vi "Counter - Read Encoder (Continuous Clock).vi"() -> ()   [LabVIEW 2017]
doc: "This example demonstrates how to use a counter input along with an external clock to continually sample the angular position measured from an encoder.\n\nFor instructions on how to connect your signals to the DAQ device, refer to your device documentation."
uses:
  <vilib>/Utility/error.llb/DialogType.ctl
  <vilib>/DAQmx/read.llb/DAQmx Read (Counter 1D DBL 1Chan NSamp).vi
  <vilib>/DAQmx/read.llb/DAQmx Read (Analog 2D DBL NChan NSamp).vi
  <vilib>/Analysis/baseanly.llb/Mean (DBL).vi
  <vilib>/DAQmx/create/channels.llb/DAQmx Create Channel (CI-Position-Linear Encoder).vi
  <vilib>/DAQmx/configure/timing.llb/DAQmx Timing (Sample Clock).vi
  <vilib>/DAQmx/create/channels.llb/DAQmx Create Channel (AI-Voltage-Basic).vi
  <vilib>/DAQmx/miscellaneous.llb/DAQmx Fill In Error Info.vi
  <resource>/objmgr/daqmx.rc
  <vilib>/Analysis/NI_AALBase.lvlib
panel:
  out "Array":dbl[](array[numeric])
  in  "minimum value":dbl=-5.0 format="%0.2f"
  in  "maximum value":dbl=5.0 format="%0.2f"
  in  "Coils":tag="PXI1Slot2/ai0:5"
  out "SampClk.Rate":dbl=1000.0
  in  "initial position":dbl
  in  "distance per pulse":dbl=0.001
  in  "Z Index Terminal":tag="PFI9"
  in  "Z Index Enable":bool
  in  "B Input Terminal":tag="PFI10"
  in  "A Input Terminal":tag="PFI8"
  in  "Counter":tag="PXI1Slot2/ctr0"
  out "Acquired Data":dbl[](array[numeric])
  in  "Stop":bool
  in  "Samples per Loop":i32=1
  in  "Sample Rate":dbl=10.0
  in  "Sample Clock Source":tag="PFI0"
  # "Channel Settings"
  # "Acquired Data"
  # "Timing Settings"
  # "Trigger Settings"
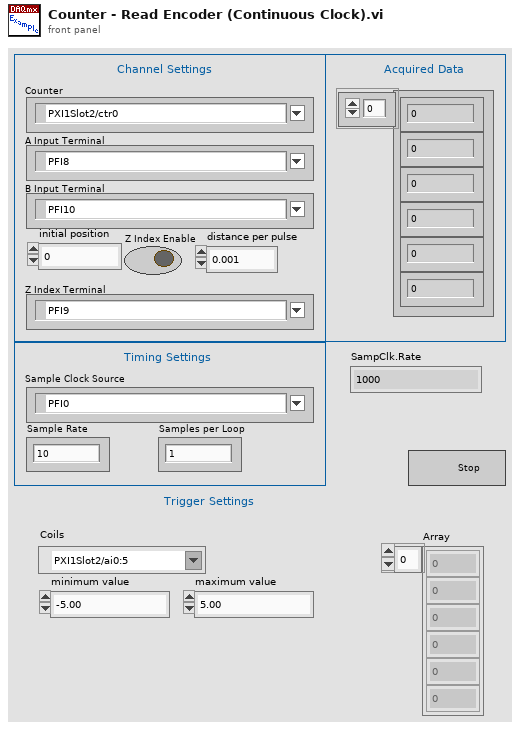
[diagram p1: front panel]
types:
  T1 = typedef "DialogType.ctl" = u16
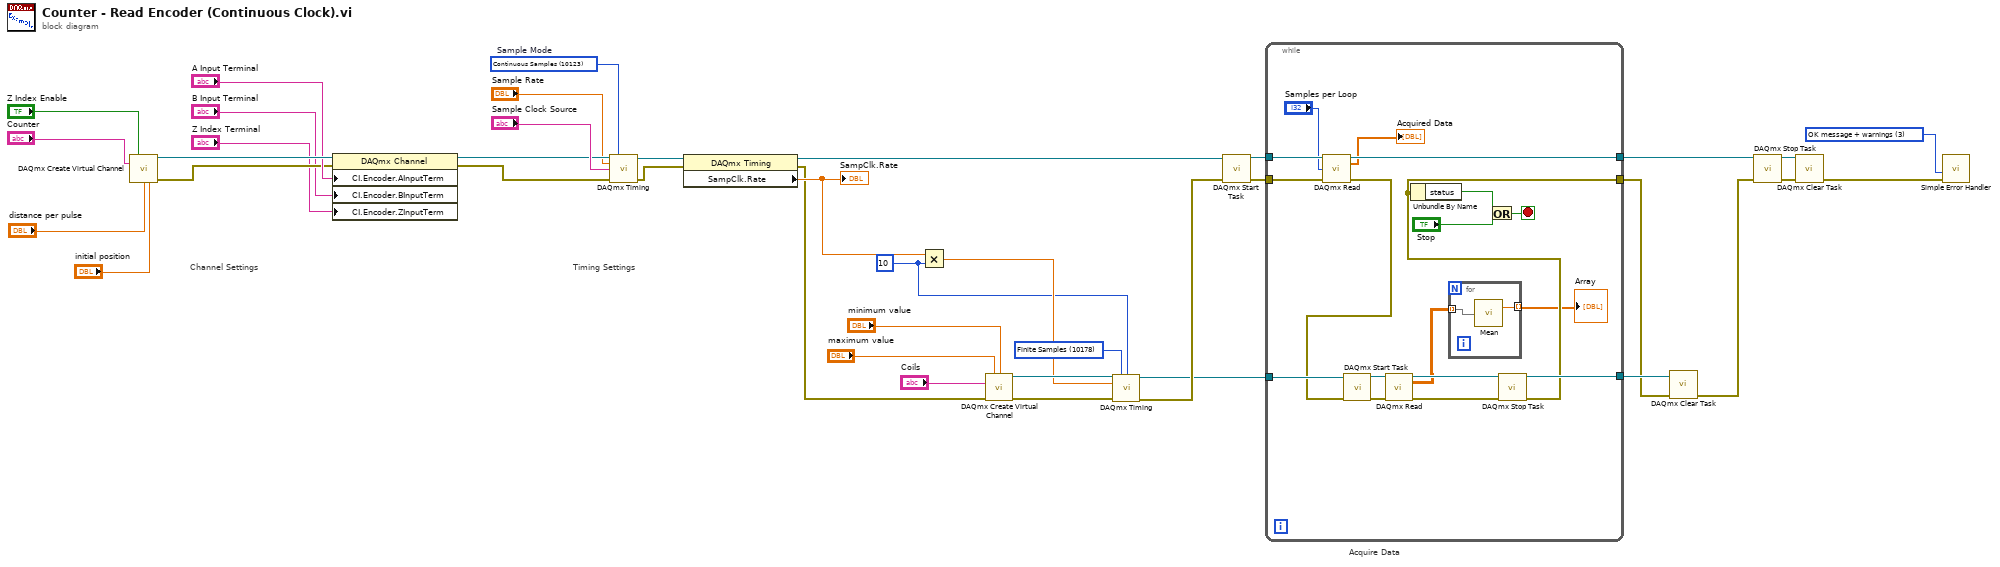
[diagram p0: block diagram]
diagram:
  w7 = 10178 items=["Finite Samples"=10178, "Continuous Samples"=10123, "Hardware Timed Single Point"=12522] ("sample mode")
  w8 = 10
  w21 = T1 3 items=["no dialog", "OK message", "continue or stop message", "OK message + warnings", "continue/stop + warnings"] ("type of dialog (OK msg:1)")
  w39 = 10123 items=["Finite Samples"=10178, "Continuous Samples"=10123, "Hardware Timed Single Point"=12522]  # Sample Mode
  # "Acquire Data"
  # "Timing Settings"
  # "Channel Settings"
  n1 = call-poly <vilib>:"DAQmx Create Virtual Channel.vi"("z index enable"="Z Index Enable", "counter"="Counter", "distance per pulse"="distance per pulse", "initial position"="initial position") -> ("task out"=w32:refnum<k21>, "error out"=w30:errorcluster)  [unwired: 10 in]
  n2 = property class="DAQmx Channel"(reference=w32, error in=w30, "CI.Encoder.AInputTerm"="A Input Terminal", "CI.Encoder.BInputTerm"="B Input Terminal", "CI.Encoder.ZInputTerm"="Z Index Terminal") -> (reference out=w26:refnum<k21>, error out=w25:errorcluster)
  n3 = call-poly <vilib>:"DAQmx Timing.vi"("task/channels in"=w26, "sample mode"=w39, "rate"="Sample Rate", "source"="Sample Clock Source", "error in"=w25) -> ("task out"=w34:refnum<k21>, "error out"=w18:errorcluster)  [unwired: 9 in]
  n4 = property class="DAQmx Timing"(reference=w34, error in=w18) -> (reference out=w17:refnum<k21>, error out=w5:errorcluster, "SampClk.Rate"=w10:dbl)
  "SampClk.Rate" <- w10
  n5 = Multiply(x=w10, y=w8) -> (x*y=w9:dbl)
  n6 = call-poly <vilib>:"DAQmx Create Virtual Channel.vi"("maximum value"="maximum value", "minimum value"="minimum value", "physical channels"="Coils", "error in"=w5) -> ("task out"=w13:refnum<k21>, "error out"=w12:errorcluster)  [unwired: 10 in]
  n7 = call-poly <vilib>:"DAQmx Timing.vi"("task/channels in"=w13, "sample mode"=w7, "samples per channel"=w8, "rate"=w9, "error in"=w12) -> ("task out"=w4:refnum<k21>, "error out"=w6:errorcluster)  [unwired: 9 in]
  n8 = call <vilib>:"DAQmx Start Task.vi"("task/channels in"=w17, "error in"=w6) -> ("task out"=w38:refnum<k21>, "error out"=w37:errorcluster)  [unwired: 12 in]
  n9 = while {
    tunnel: w38 -> [w57]
    tunnel: w37 -> [w56]
    tunnel: [w42] -> w2
    tunnel: [w54] -> w24
    tunnel: w4 -> [w49]
    tunnel: [w44] -> w3
    stop <- w55 stop-if-true
    n10 = call-poly <vilib>:"DAQmx Read.vi"("task/channels in"=w57, "number of samples per channel"="Samples per Loop", "error in"=w56) -> ("task out"=w54:refnum<k21>, "data"=→"Acquired Data":dbl[], "error out"=w43:errorcluster)  [unwired: 10 in]
    n11 = call <vilib>:"DAQmx Start Task.vi"("task/channels in"=w49, "error in"=w43) -> ("task out"=w47:refnum<k21>, "error out"=w48:errorcluster)  [unwired: 12 in]
    n12 = call-poly <vilib>:"DAQmx Read.vi"("task/channels in"=w47, "error in"=w48) -> ("task out"=w46:refnum<k21>, "data"=w41:dbl[][], "error out"=w45:errorcluster)  [unwired: 11 in]
    n13 = for {
      tunnel: w41 -> [w59] mode=indexing
      tunnel: [w58] -> w40 mode=indexing
      n14 = call-poly <vilib>:"Mean.vi"("X"=w59) -> ("mean"=w58:dbl)  [unwired: 1 out]
    }
    "Array" <- w40
    n15 = call <vilib>:"DAQmx Stop Task.vi"("task/channels in"=w46, "error in"=w45) -> ("task out"=w44:refnum<k21>, "error out"=w42:errorcluster)  [unwired: 12 in]
    n16 = Unbundle By Name(w42) -> ("status"=w53:bool)
    n17 = Or(x=w53, y="Stop") -> (x .or. y?=w55:bool)
  }
  n18 = call <vilib>:"DAQmx Clear Task.vi"("task in"=w3, "error in"=w2) -> ("error out"=w1:errorcluster)  [unwired: 13 in]
  n19 = call <vilib>:"DAQmx Stop Task.vi"("task/channels in"=w24, "error in"=w1) -> ("task out"=w22:refnum<k21>, "error out"=w23:errorcluster)  [unwired: 12 in]
  n20 = call <vilib>:"DAQmx Clear Task.vi"("task in"=w22, "error in"=w23) -> ("error out"=w36:errorcluster)  [unwired: 13 in]
  n21 = call <vilib>:"Simple Error Handler.vi"("type of dialog (OK msg:1)"=w21, "error in (no error)"=w36) -> ()  [unwired: 3 in, 5 out]
